vi "move large data(wip) for real.vi"() -> ()   [LabVIEW 2020, in "Data.PG.lvclass"]
uses:
  Data.PG.lvclass
panel:
  out "standard error":string
  out "standard output":string="Microsoft Windows [Version 10.0.18363.900]\r\n(c) 2019 Microsoft Corporation. All rights reserved.\r\n\r\nC:\\>C:\\Users\\ansom_voodoo\\Desktop\\temporary.bat\r\nCOPY 1\r\nPress any key to continue . . . \r\n\r\nC:\\>"
  in  "password":string="711elvis"
  in  "username":string="phil"
  in  "table":string="llab_hello"
  in  "database":string="postgres"
  in  "port":string="5432"
  in  "host":string="ec2-18-220-14-159.us-east-2.compute.amazonaws.com"
  in  "Path to data csv":path=path "C:/Users/ansom_voodoo/Desktop/test.csv"
  in  "path okay for temporary file":path=path "C:/Users/ansom_voodoo/Desktop"
  in  "OK":bool
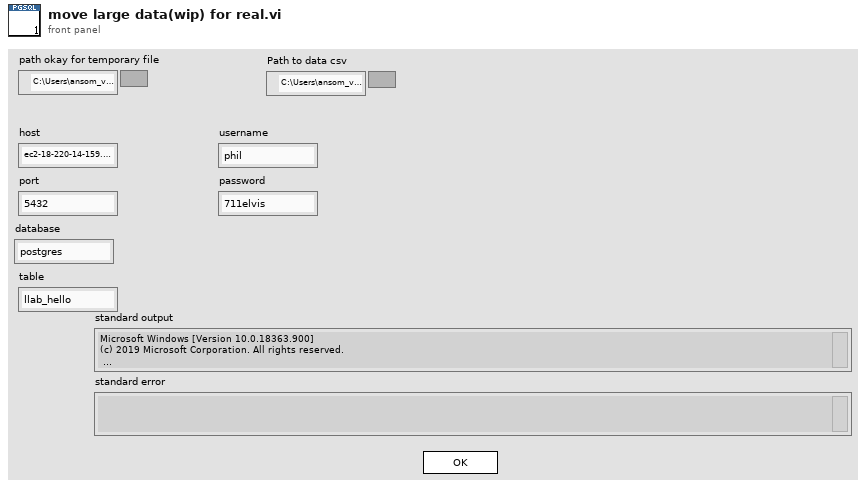
[diagram p1: front panel]
types:
  T1 = enum32{"Invalid", "Standard", "Closed", "Hidden", "Minimized", "Maximized"}
  T2 = enum32{"invalid app kind", "Development System", "Run Time System", "Student Edition", "Embedded LabVIEW", "Evaluation", "Custom"}
  T3 = cluster{"Core":cluster{"Current VI Reference":refnum<vi>, "Close Panel on Exit?":bool}, "Path to temp file":path, "name of temp file":string, "path to csv data":path, "host":string, "username":string, "password":string, "database":string, "port":string, "table name":string, "path to run":path}
  T4 = cluster{"Current VI Reference":refnum<vi>, "Close Panel on Exit?":bool}
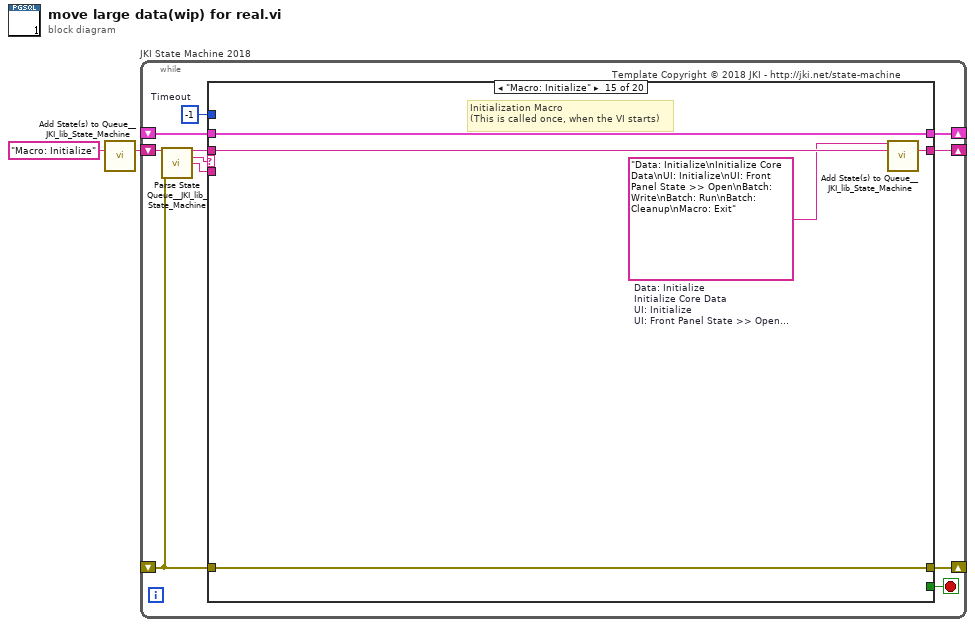
[diagram p0: block diagram]
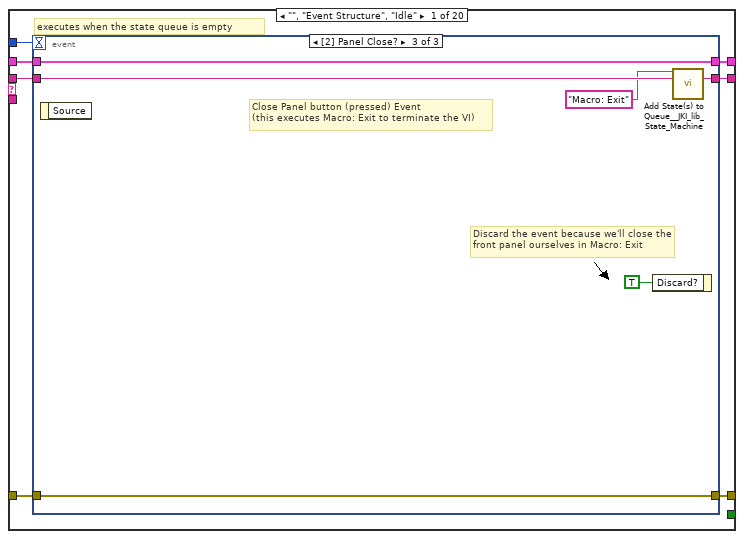
[diagram p2: hidden frame]
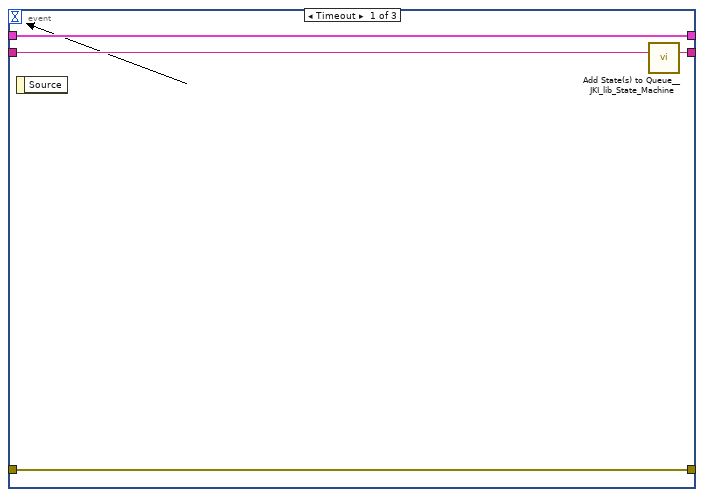
[diagram p3: hidden frame]
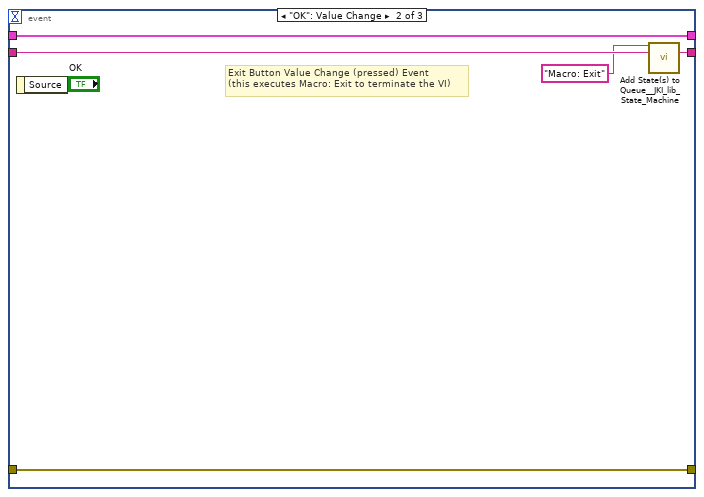
[diagram p4: hidden frame]
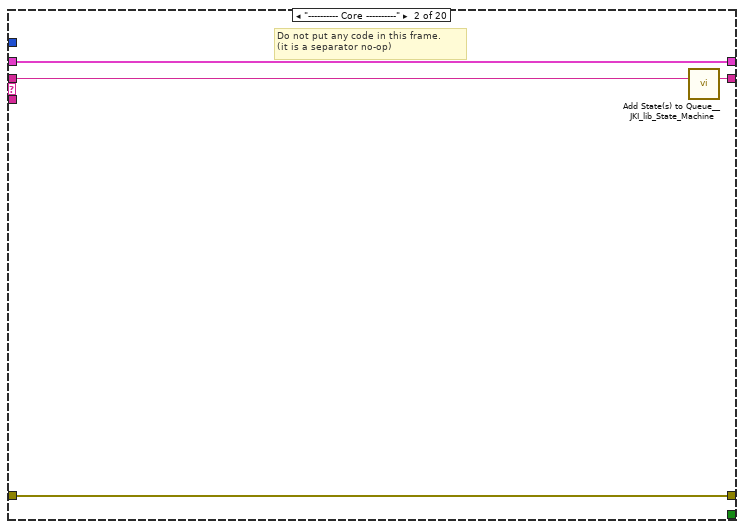
[diagram p5: hidden frame]
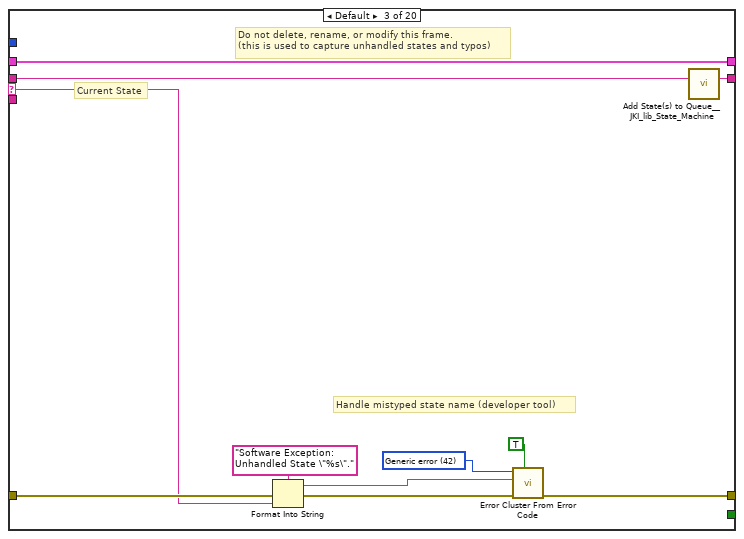
[diagram p6: hidden frame]
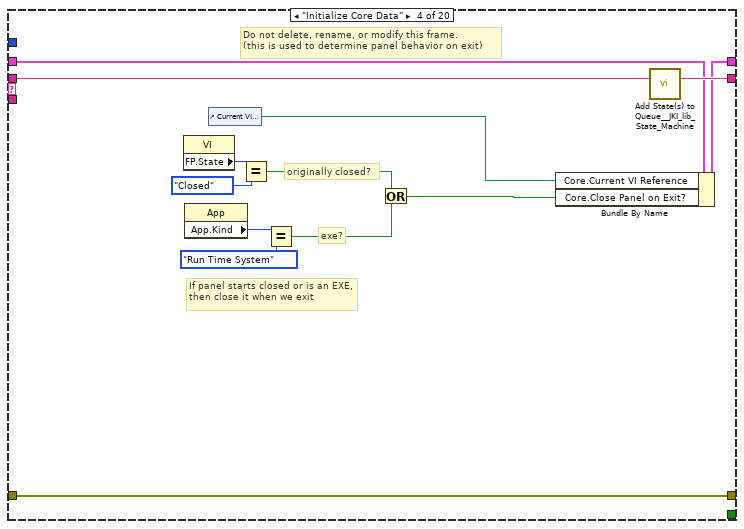
[diagram p7: hidden frame]
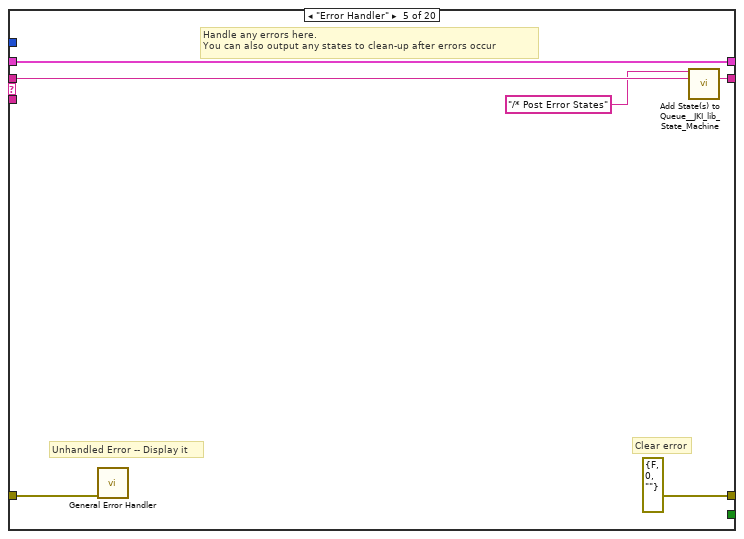
[diagram p8: hidden frame]
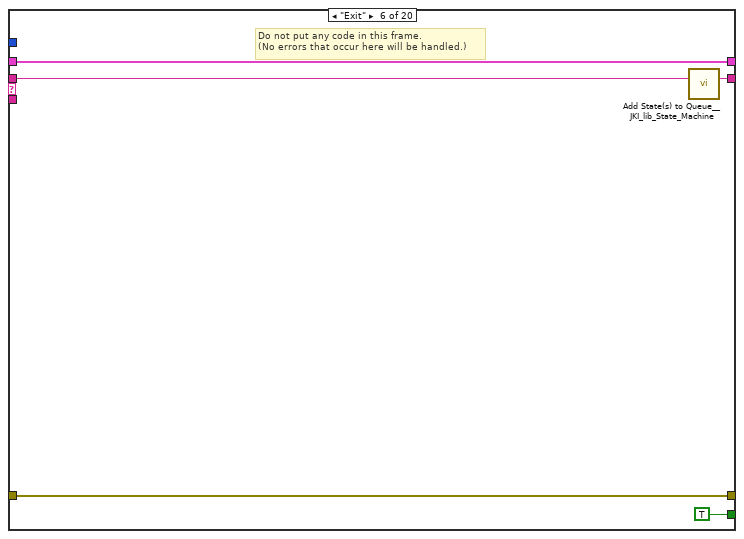
[diagram p9: hidden frame]
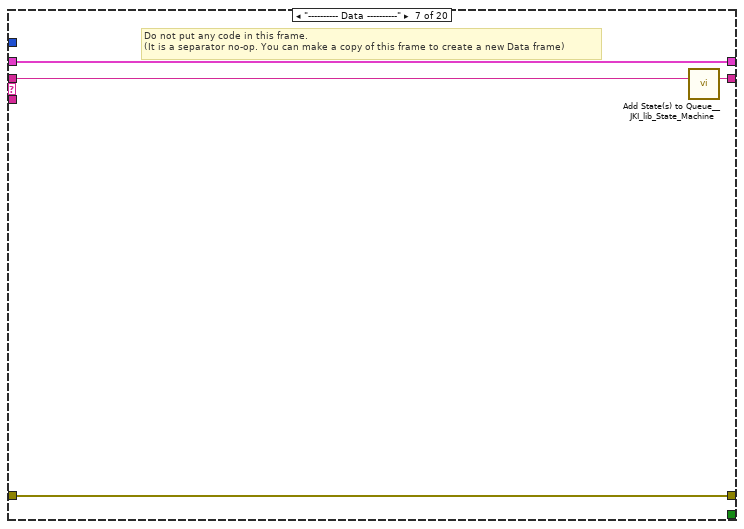
[diagram p10: hidden frame]
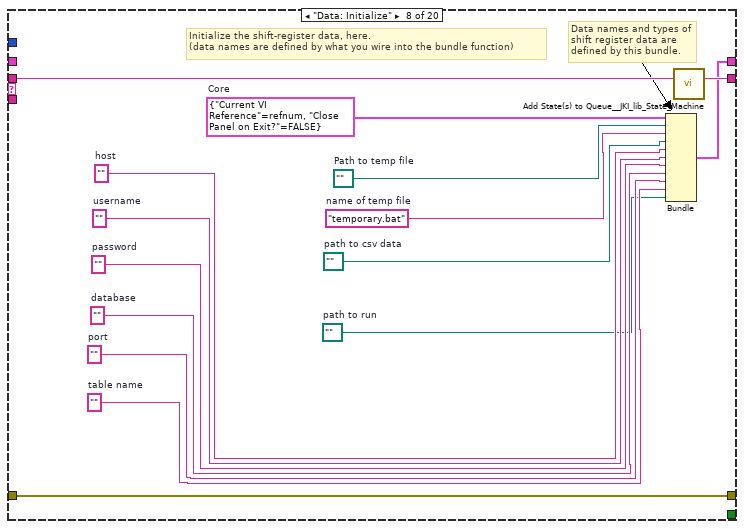
[diagram p11: hidden frame]
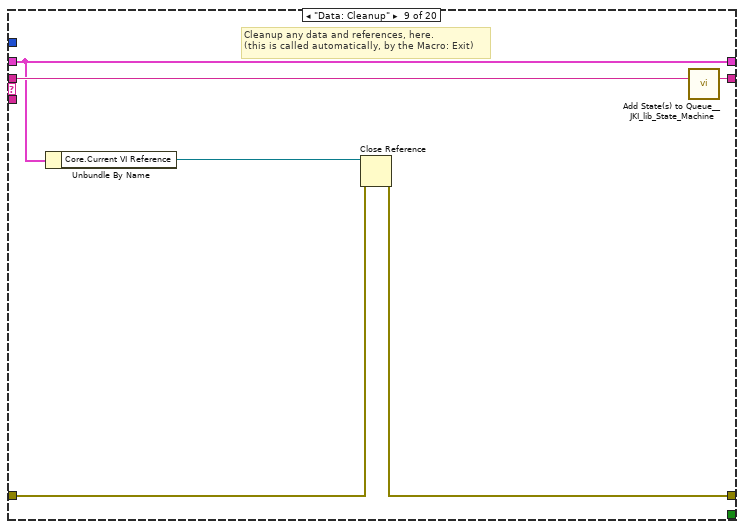
[diagram p12: hidden frame]
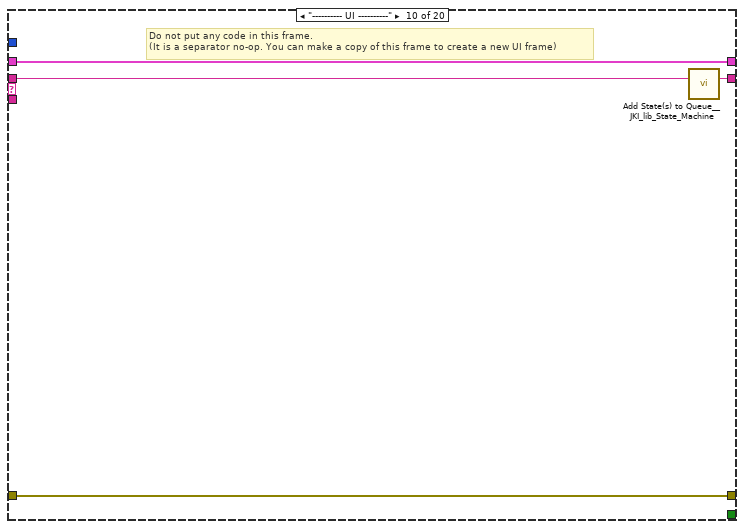
[diagram p13: hidden frame]
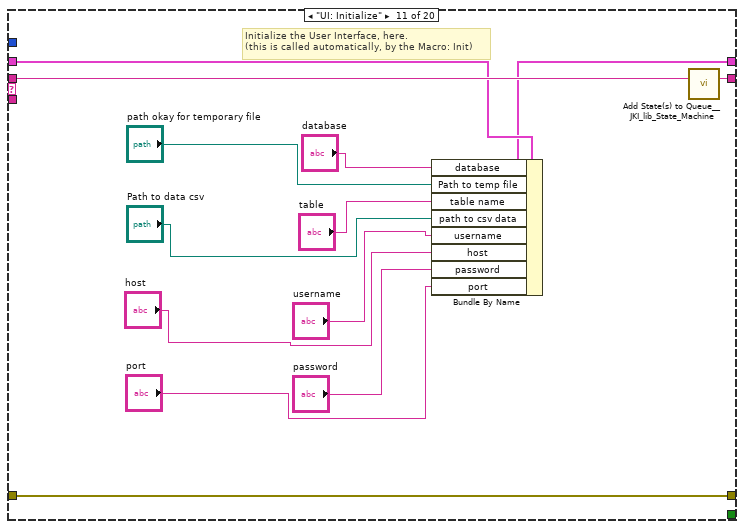
[diagram p14: hidden frame]
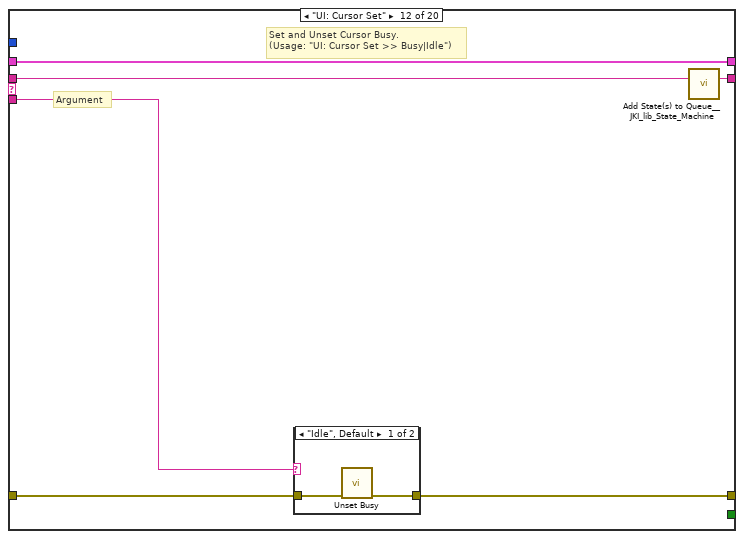
[diagram p15: hidden frame]
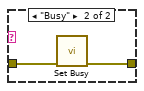
[diagram p16: hidden frame]
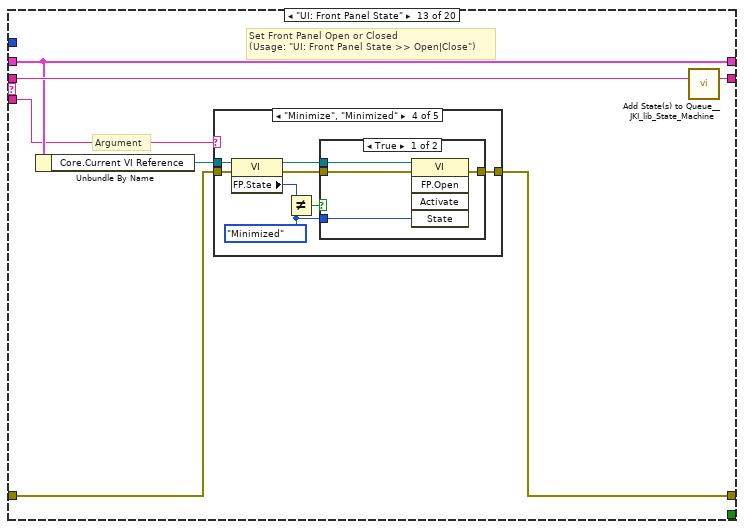
[diagram p17: hidden frame]
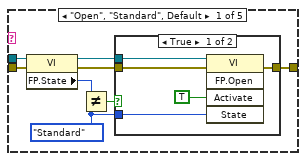
[diagram p18: hidden frame]
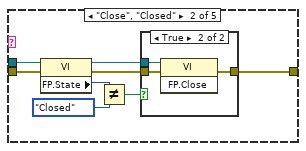
[diagram p20: hidden frame]
diagram:
  n1 = call <vilib>:"Add State(s) to Queue__JKI_lib_State_Machine.vi"("State(s) in (\"\")"="Macro: Initialize") -> ("States Out"=w2:string)  [unwired: 14 in]
  n2 = while "JKI State Machine 2018" {
    shift-right: [w6] -> _
    shift-left: _ -> [w5]
    shift-right: [w9] -> _
    shift-left: _ -> [w3]
    shift-right: [w8] -> _
    shift-left: w2 -> [w10]
    stop <- w7 stop-if-true
    w4 = -1  # Timeout
    # "Template Copyright © 2018 JKI - http://jki.net/state-machine"
    n3 = call <vilib>:"Parse State Queue__JKI_lib_State_Machine.vi"("State Queue"=w10, "Error In (no error)"=w3) -> ("Remaining States"=w12:string, "Current State"=w13:string, "Arguments"=w11:string)  [unwired: 11 in]
    n4 = case shown="\"Macro: Initialize\"" w13 {
      selector: w13 -> [_ _ w40 _ _ _ _ _ _ _ _ _ _ _ _ _ _ _ _ _]
      tunnel: w12 -> [w20 w39 w44 w63 w69 w74 w78 w93 w99 w103 w116 w122 w133 w202 w207 w217 w221 w240 w253 w258]
      tunnel: w11 -> [_ _ _ _ _ _ _ _ _ _ _ w117 w127 _ _ _ _ _ _ _]
      tunnel: w5 -> [w18 w36 w42 w56 w66 w72 w75 _ w94 w100 w113 w120 w129 w199 w204 w214 w218 w232 w250 w255]
      tunnel: [w17 w37 w46 w60 errorcluster {"status"=FALSE, "code"=0, "source"=""} ("error out") w71 w76 w90 w95 w101 w114 w118 w130 w200 w205 w215 w219 w238 w251 w256] -> w9
      tunnel: w3 -> [w16 w37 w45 w60 w65 w71 w76 w90 w96 w101 w114 w119 w131 w200 w205 w215 w219 w238 w251 w256]
      tunnel: [w19 w38 w43 w62 w68 w73 w77 w92 w98 w102 w115 w121 w132 w201 w206 w216 w220 w239 w252 w257] -> w8
      tunnel: [_ _ _ _ _ TRUE _ _ _ _ _ _ _ _ _ _ _ _ _ _] -> w7
      tunnel: [w15 w36 w42 w61 w66 w72 w75 w91 w94 w100 w112 w120 w129 w199 w204 w214 w218 w235 w250 w255] -> w6
      tunnel: w4 -> [w14 _ _ _ _ _ _ _ _ _ _ _ _ _ _ _ _ _ _ _]
      frame "", "Event Structure", "Idle" {
        # "executes when the state queue is empty"
        n5 = event shown="[2] Panel Close?" {
          selector: _ -> [_ _ _]
          dyn-events: _ -> [_ _ _]
          timeout: w14 -> [_ _ _]
          tunnel: w20 -> [w24 w29 w35]
          tunnel: [w23 w28 w34] -> w19
          tunnel: w18 -> [w21 w26 w32]
          tunnel: [w22 w27 w33] -> w17
          tunnel: w16 -> [w22 w27 w33]
          tunnel: [w21 w26 w32] -> w15
          event Timeout {
            n6 = event-data() -> ()  [unwired: 1 in, 1 out]
            n7 = call <vilib>:"Add State(s) to Queue__JKI_lib_State_Machine.vi"("State(s) in (\"\")"=w24) -> ("States Out"=w23:string)  [unwired: 14 in]
          }
          event "OK": Value Change {
            # "Exit Button Value Change (pressed) Event\n(this executes Macro: Exit to terminate the VI)"
            n8 = event-data() -> ()  [unwired: 1 in, 1 out]
            n9 = call <vilib>:"Add State(s) to Queue__JKI_lib_State_Machine.vi"("State(s) in Front (\"\")"="Macro: Exit", "State(s) in (\"\")"=w29) -> ("States Out"=w28:string)  [unwired: 13 in]
          }
          event Panel Close? {
            # "Discard the event because we'll close the front panel ourselves in Macro: Exit"
            # "Close Panel button (pressed) Event\n(this executes Macro: Exit to terminate the VI)"
            n10 = event-data() -> ()  [unwired: 1 in, 1 out]
            n11 = event-data("Discard?"=TRUE) -> ()  [unwired: 1 in, 1 out]
            n12 = call <vilib>:"Add State(s) to Queue__JKI_lib_State_Machine.vi"("State(s) in Front (\"\")"="Macro: Exit", "State(s) in (\"\")"=w35) -> ("States Out"=w34:string)  [unwired: 13 in]
          }
        }
      }
      frame "---------- Core ----------" {
        # "Do not put any code in this frame.\n(it is a separator no-op)"
        n13 = call <vilib>:"Add State(s) to Queue__JKI_lib_State_Machine.vi"("State(s) in (\"\")"=w39) -> ("States Out"=w38:string)  [unwired: 14 in]
      }
      frame Default {
        w49 = 42 items=["No error", "Argument error", "Memory is full", "Out of zone", "End of file", "File already open", "Generic file I/O error", "File not found", "File permission error", "Disk is full", "Duplicate path", "Too many files open", "System feature not enabled", "Resource file not found", "Cannot add resource", "Resource not found", "Image not found", "Image memory error", "Pen does not exist", "Config type invalid", "Config token not found", "Config parse error", "Config memory error", "Bad external code format", "Bad external code offset", "External code not present", "Null window", "Destroy window error", "Null menu", "Print aborted", "Bad print record", "Print driver error", "Windows error during printing", "Memory error during printing", "Print dialog error", "Generic print error", "Invalid device refnum", "Device not found", "Device parameter error", "Device unit error", "Cannot open device", "Device call aborted", "Generic error", "Cancelled by user", "Object ID too low", "Object ID too high", "Object not in heap", "Unknown heap", "Unknown object (invalid DefProc)", "Unknown object (DefProc not in table)", "Message out of range", "Invalid (null) method", "Unknown message", "Manager call not supported", "Bad address", "Network operation in progress", "Network operation timed out", "Connection is busy", "Network attribute not supported", "Network error", "Address in use", "System out of memory", "Connection aborted", "Connection refused", "Not connected", "Already connected", "Connection closed", "Initialization error (interapplication manager)", "Bad occurrence", "Wait on unbound occurrence handler", "Occurrence queue overflow", "Datalog type conflict", "Unused", "Unrecognized type (interapplication manager)", "Memory corrupt", "Failed to make temporary DLL", "Old CIN version", "Drag socket not found", "Failed to load drop-object", "Failed to register OLE object", "Failed to release OLE object", "Format specifier type mismatch", "Unknown format specifier", "Too few format specifiers", "Too many format specifiers", "Scan failed", "Newer CIN version", "Error converting to variant", "Runtime menu error", "Password tampered", "Variant attribute not found", "Incompatible variant data type", "Event data is not available", "Event Store is not present", "Occurrence is not found", "Event Queue is not created", "Event info is not available", "Refnum passed is NULL", "Error retrieving Class GUID", "Error retrieving CoClass GUID", "Error retrieving TypeLib GUID.", "Bad built application magic bytes.", "Specific driver is different from the specific driver associated with the Logical Name.", "There is no session opened to the class driver.", "Max Error", "MAX - Error with config objects", "MAX - Error loading configuration", "MAX - Group not supported"]
        # "Current State"
        # "Do not delete, rename, or modify this frame.\n(this is used to capture unhandled states and typos)"
        # "Handle mistyped state name (developer tool)"
        n14 = Format Into String(format string="Software Exception: Unhandled State \"%s\"." ("message"), error in=w45, w40) -> (resulting string=w48:string, error out=w47:errorcluster)  [unwired: 1 in]
        n15 = call <vilib>:"Error Cluster From Error Code.vi"("show call chain? (False)"=TRUE, "error in (no error)"=w47, "error message (\"\")"=w48, "error code (0)"=w49) -> ("error out"=w46:errorcluster)  [unwired: 5 in]
        n16 = call <vilib>:"Add State(s) to Queue__JKI_lib_State_Machine.vi"("State(s) in (\"\")"=w44) -> ("States Out"=w43:string)  [unwired: 14 in]
      }
      frame "Initialize Core Data" {
        # "Do not delete, rename, or modify this frame.\n(this is used to determine panel behavior on exit)"
        # "originally closed?"
        # "exe?"
        # "If panel starts closed or is an EXE, then close it when we exit"
        n17 = property class="VI"() -> ("FP.State"=w53:T1)  [unwired: 2 in, 2 out]
        n18 = property class="App"() -> ("App.Kind"=w59:T2)  [unwired: 2 in, 2 out]
        n19 = control-ref of="Current VI Reference"() -> (w54:refnum<vi>)
        n20 = Equal?(x=w53, y=T1."Closed" ("Front Panel Window:State")) -> (x = y?=w51:bool)
        n21 = Equal?(x=w59, y=T2."Run Time System" ("Application:Kind")) -> (x = y?=w57:bool)
        n22 = Or(x=w51, y=w57) -> (x .or. y?=w55:bool)
        n23 = Bundle By Name(cluster=w56, "Core.Current VI Reference"=w54, "Core.Close Panel on Exit?"=w55) -> (w61:T3)
        n24 = call <vilib>:"Add State(s) to Queue__JKI_lib_State_Machine.vi"("State(s) in (\"\")"=w63) -> ("States Out"=w62:string)  [unwired: 14 in]
      }
      frame "Error Handler" {
        # "Unhandled Error -- Display it"
        # "Handle any errors here.\nYou can also output any states to clean-up after errors occur"
        # "Clear error"
        n25 = call <vilib>:"General Error Handler.vi"("error in (no error)"=w65) -> ()  [unwired: 10 in, 5 out]
        n26 = call <vilib>:"Add State(s) to Queue__JKI_lib_State_Machine.vi"("State(s) in Front (\"\")"="/* Post Error States", "State(s) in (\"\")"=w69) -> ("States Out"=w68:string)  [unwired: 13 in]
      }
      frame "Exit" {
        # "Do not put any code in this frame.\n(No errors that occur here will be handled.)"
        n27 = call <vilib>:"Add State(s) to Queue__JKI_lib_State_Machine.vi"("State(s) in (\"\")"=w74) -> ("States Out"=w73:string)  [unwired: 14 in]
      }
      frame "---------- Data ----------" {
        # "Do not put any code in this frame.\n(It is a separator no-op. You can make a copy of this frame to create a new Data frame)"
        n28 = call <vilib>:"Add State(s) to Queue__JKI_lib_State_Machine.vi"("State(s) in (\"\")"=w78) -> ("States Out"=w77:string)  [unwired: 14 in]
      }
      frame "Data: Initialize" {
        w79 = path ""  # path to run
        w80 = ""  # table name
        w81 = ""  # port
        w82 = ""  # database
        w83 = ""  # password
        w84 = ""  # username
        w85 = ""  # host
        w86 = path ""  # path to csv data
        w87 = "temporary.bat"  # name of temp file
        w88 = path ""  # Path to temp file
        w89 = T4 {"Current VI Reference"=refnum, "Close Panel on Exit?"=FALSE}  # Core
        # "Data names and types of shift register data are defined by this bundle."
        # "Initialize the shift-register data, here.\n(data names are defined by what you wire into the bundle function)"
        n29 = Bundle("Core"=w89, "Path to temp file"=w88, "name of temp file"=w87, "path to csv data"=w86, "host"=w85, "username"=w84, "password"=w83, "database"=w82, "port"=w81, "table name"=w80, "path to run"=w79) -> (w91:T3)  [unwired: 1 in]
        n30 = call <vilib>:"Add State(s) to Queue__JKI_lib_State_Machine.vi"("State(s) in (\"\")"=w93) -> ("States Out"=w92:string)  [unwired: 14 in]
      }
      frame "Data: Cleanup" {
        # "Cleanup any data and references, here.\n(this is called automatically, by the Macro: Exit)"
        n31 = Unbundle By Name(w94) -> ("Core.Current VI Reference"=w97:refnum<vi>)
        n32 = Close Reference(reference=w97, error in (no error)=w96) -> (error out=w95:errorcluster)
        n33 = call <vilib>:"Add State(s) to Queue__JKI_lib_State_Machine.vi"("State(s) in (\"\")"=w99) -> ("States Out"=w98:string)  [unwired: 14 in]
      }
      frame "---------- UI ----------" {
        # "Do not put any code in this frame.\n(It is a separator no-op. You can make a copy of this frame to create a new UI frame)"
        n34 = call <vilib>:"Add State(s) to Queue__JKI_lib_State_Machine.vi"("State(s) in (\"\")"=w103) -> ("States Out"=w102:string)  [unwired: 14 in]
      }
      frame "UI: Initialize" {
        # "Initialize the User Interface, here.\n(this is called automatically, by the Macro: Init)"
        n35 = Bundle By Name(cluster=w113, "database"="database", "Path to temp file"="path okay for temporary file", "table name"="table", "path to csv data"="Path to data csv", "username"="username", "host"="host", "password"="password", "port"="port") -> (w112:T3)
        n36 = call <vilib>:"Add State(s) to Queue__JKI_lib_State_Machine.vi"("State(s) in (\"\")"=w116) -> ("States Out"=w115:string)  [unwired: 14 in]
      }
      frame "UI: Cursor Set" {
        # "Argument"
        # "Set and Unset Cursor Busy.\n(Usage: \"UI: Cursor Set >> Busy|Idle\")"
        n37 = case shown="\"Idle\", Default" w117 {
          tunnel: w119 -> [w124 w126]
          tunnel: [w123 w125] -> w118
          frame "Idle", Default {
            n38 = call <vilib>:"Unset Busy.vi"("error in (no error)"=w124) -> ("error out"=w123:errorcluster)  [unwired: 10 in]
          }
          frame "Busy" {
            n39 = call <vilib>:"Set Busy.vi"("error in (no error)"=w126) -> ("error out"=w125:errorcluster)  [unwired: 9 in, 1 out]
          }
        }
        n40 = call <vilib>:"Add State(s) to Queue__JKI_lib_State_Machine.vi"("State(s) in (\"\")"=w122) -> ("States Out"=w121:string)  [unwired: 14 in]
      }
      frame "UI: Front Panel State" {
        # "Argument"
        # "Set Front Panel Open or Closed\n(Usage: \"UI: Front Panel State >> Open|Close\")"
        n41 = Unbundle By Name(w129) -> ("Core.Current VI Reference"=w128:refnum<vi>)
        n42 = case shown="\"Minimize\", \"Minimized\"" w127 {
          tunnel: w131 -> [w139 w154 w165 w178 w191]
          tunnel: [w141 w155 w167 w180 w193] -> w130
          tunnel: w128 -> [w140 w152 w166 w179 w192]
          frame "Open", "Standard", Default {
            w134 = T1."Standard" ("State")
            n43 = property class="VI"(reference=w140, error in=w139) -> (reference out=w137:refnum<vi>, error out=w138:errorcluster, "FP.State"=w136:T1)
            n44 = Not Equal?(x=w136, y=w134) -> (x != y?=w135:bool)
            n45 = case shown="True" w135 {
              tunnel: [w145 w147] -> w141
              tunnel: w138 -> [w144 w147]
              tunnel: w137 -> [w143 _]
              tunnel: w134 -> [w142 _]
              frame True {
                n46 = invoke class="VI" method="FP.Open"(reference=w143, error in=w144, "Activate"=TRUE, "State"=w142) -> (error out=w145:errorcluster)  [unwired: 1 in, 4 out]
              }
              frame False {
              }
            }
          }
          frame "Close", "Closed" {
            n47 = property class="VI"(reference=w152, error in=w154) -> (reference out=w151:refnum<vi>, error out=w153:errorcluster, "FP.State"=w149:T1)
            n48 = Not Equal?(x=w149, y=T1."Closed" ("Front Panel Window:State")) -> (x != y?=w148:bool)
            n49 = case shown="True" w148 {
              tunnel: [w156 w159] -> w155
              tunnel: w153 -> [w156 w158]
              tunnel: w151 -> [_ w157]
              frame False {
              }
              frame True {
                n50 = invoke class="VI" method="FP.Close"(reference=w157, error in=w158) -> (error out=w159:errorcluster)  [unwired: 1 in, 2 out]
              }
            }
          }
          frame "Hidden", "Hide" {
            w160 = T1."Hidden" ("State")
            n51 = property class="VI"(reference=w166, error in=w165) -> (reference out=w163:refnum<vi>, error out=w164:errorcluster, "FP.State"=w162:T1)
            n52 = Not Equal?(x=w162, y=w160) -> (x != y?=w161:bool)
            n53 = case shown="True" w161 {
              tunnel: [w171 w172] -> w167
              tunnel: w164 -> [w170 w172]
              tunnel: w163 -> [w169 _]
              tunnel: w160 -> [w168 _]
              frame True {
                n54 = invoke class="VI" method="FP.Open"(reference=w169, error in=w170, "State"=w168) -> (error out=w171:errorcluster)  [unwired: 2 in, 4 out]
              }
              frame False {
              }
            }
          }
          frame "Minimize", "Minimized" {
            w173 = T1."Minimized" ("State")
            n55 = property class="VI"(reference=w179, error in=w178) -> (reference out=w176:refnum<vi>, error out=w177:errorcluster, "FP.State"=w175:T1)
            n56 = Not Equal?(x=w175, y=w173) -> (x != y?=w174:bool)
            n57 = case shown="True" w174 {
              tunnel: [w184 w185] -> w180
              tunnel: w177 -> [w183 w185]
              tunnel: w176 -> [w182 _]
              tunnel: w173 -> [w181 _]
              frame True {
                n58 = invoke class="VI" method="FP.Open"(reference=w182, error in=w183, "State"=w181) -> (error out=w184:errorcluster)  [unwired: 2 in, 4 out]
              }
              frame False {
              }
            }
          }
          frame "Maximize", "Maximized" {
            w186 = T1."Maximized" ("State")
            n59 = property class="VI"(reference=w192, error in=w191) -> (reference out=w189:refnum<vi>, error out=w190:errorcluster, "FP.State"=w188:T1)
            n60 = Not Equal?(x=w188, y=w186) -> (x != y?=w187:bool)
            n61 = case shown="True" w187 {
              tunnel: [w197 w198] -> w193
              tunnel: w190 -> [w196 w198]
              tunnel: w189 -> [w195 _]
              tunnel: w186 -> [w194 _]
              frame True {
                n62 = invoke class="VI" method="FP.Open"(reference=w195, error in=w196, "State"=w194) -> (error out=w197:errorcluster)  [unwired: 2 in, 4 out]
              }
              frame False {
              }
            }
          }
        }
        n63 = call <vilib>:"Add State(s) to Queue__JKI_lib_State_Machine.vi"("State(s) in (\"\")"=w133) -> ("States Out"=w132:string)  [unwired: 14 in]
      }
      frame "---------- Macro ----------" {
        # "Do not put any code in this frame.\n(It is a separator no-op. You can make a copy of this frame to create a new Macro frame)"
        n64 = call <vilib>:"Add State(s) to Queue__JKI_lib_State_Machine.vi"("State(s) in (\"\")"=w202) -> ("States Out"=w201:string)  [unwired: 14 in]
      }
      frame "Macro: Initialize" {
        w203 = "Data: Initialize\nInitialize Core Data\nUI: Initialize\nUI: Front Panel State >> Open\nBatch: Write\nBatch: Run\nBatch: Cleanup\nMacro: Exit"  # Data: Initialize Initialize Core Data UI: Initialize UI: Front Panel State >> Open Batch: Write Batch: Run Batch: Cleanup Macro: Exit
        # "Initialization Macro\n(This is called once, when the VI starts)"
        n65 = call <vilib>:"Add State(s) to Queue__JKI_lib_State_Machine.vi"("State(s) in Front (\"\")"=w203, "State(s) in (\"\")"=w207) -> ("States Out"=w206:string)  [unwired: 13 in]
      }
      frame "Macro: Exit" {
        # "Exit Macro\n(This is called once, when the VI exits)"
        n66 = Unbundle By Name(w214) -> ("Core.Close Panel on Exit?"=w213:bool)
        n67 = Select(t="UI: Front Panel State >> Close", s=w213, f="") -> (s? t:f=w210:string)
        n68 = call <vilib>:"Add State(s) to Queue__JKI_lib_State_Machine.vi"("State(s) in (\"\")"=w210, "State(s) at Back (\"\")"="Data: Cleanup\nExit") -> ("States Out"=w208:string)  [unwired: 13 in]
        n69 = call <vilib>:"Add State(s) to Queue__JKI_lib_State_Machine.vi"("State(s) in Front (\"\")"=w208, "State(s) in (\"\")"=w217) -> ("States Out"=w216:string)  [unwired: 13 in]
      }
      frame "---------- Batch ----------" {
        # "Template Separator\n(You can make a copy of, or modify, this frame)"
        n70 = call <vilib>:"Add State(s) to Queue__JKI_lib_State_Machine.vi"("State(s) in (\"\")"=w221) -> ("States Out"=w220:string)  [unwired: 14 in]
      }
      frame "Batch: Write" {
        # "Template Separator\n(You can make a copy of, or modify, this frame)"
        n71 = Unbundle By Name(w232) -> ("Path to temp file"=w237:path, "name of temp file"=w236:string)
        n72 = Unbundle By Name(w232) -> ("table name"=w231:string, "path to csv data"=w230:path, "username"=w228:string, "password"=w227:string, "host"=w226:string, "port"=w225:string, "database"=w224:string)
        n73 = Build Path(base path=w237, name or relative path=w236) -> (appended path=w234:path)
        n74 = Path To String(path=w230) -> (string=w229:string)
        n75 = Bundle By Name(cluster=w232, "path to run"=w234) -> (w235:T3)
        n76 = Format Into String(format string="  %s from '%s' delimiter ',' | psql postgres://%s:%s@%s:%s/%s\nPAUSE", initial string="@ECHO OFF\necho \\copy", w231, w229, w228, w227, w226, w225, w224) -> (resulting string=w223:string)  [unwired: 1 in, 1 out]
        n77 = call <vilib>:"Add State(s) to Queue__JKI_lib_State_Machine.vi"("State(s) in (\"\")"=w240) -> ("States Out"=w239:string)  [unwired: 14 in]
        n78 = Write to Text File(file (use dialog)=w234, text=w223) -> ()  [unwired: 2 in, 3 out]
      }
      frame "Batch: Run" {
        # "Your code here.\n(You can make a copy of, or modify, this frame)"
        n79 = Unbundle By Name(w250) -> ("path to run"=w249:path)
        n80 = Path To String(path=w249) -> (string=w244:string)
        n81 = Concatenate Strings(w244, "\r\n") -> (w242:string)
        n82 = call <vilib>:"System Exec.vi"("wait until completion? (T)"=TRUE, "working directory"=path "C:/", "standard input"=w242, "command line"="cmd") -> ("standard error"=→"standard error":string, "standard output"=→"standard output":string)  [unwired: 4 in, 2 out]
        n83 = call <vilib>:"Add State(s) to Queue__JKI_lib_State_Machine.vi"("State(s) in (\"\")"=w253) -> ("States Out"=w252:string)  [unwired: 14 in]
      }
      frame "Batch: Cleanup" {
        # "Template Separator\n(You can make a copy of, or modify, this frame)"
        n84 = Unbundle By Name(w255) -> ("path to run"=w254:path)
        n85 = Delete(path (use dialog)=w254) -> ()  [unwired: 4 in, 3 out]
        n86 = call <vilib>:"Add State(s) to Queue__JKI_lib_State_Machine.vi"("State(s) in (\"\")"=w258) -> ("States Out"=w257:string)  [unwired: 14 in]
      }
    }
  }
